vi "Q1.vi"() -> ()   [LabVIEW 2019]
uses:
  <vilib>/measure/matone.llb/Extract Multiple Tone Information 1 Chan.vi
  <vilib>/measure/matone.llb/Extract Single Tone Information N Chan.vi
  <vilib>/measure/NI_MAPro.lvlib
panel:
  out "DHT <=10%":bool[](array[boolean])
  in  "stop":bool
  in  "LIGAR":bool
  in  "file path":path=path "C:/lista2.tdms"
  out "ONDA TOTAL":waveform(dbl)(graph)
  out "multiple tone information":T1(array[cluster]) {"detected phase (deg)" format="%_6g"; "detected amplitude" format="%_6p"; "detected frequency" format="%_6p"}
  out "ONDA 1":dynamicdata(graph)
  out "ONDA 3":dynamicdata(graph)
  out "ONDA 2":dynamicdata(graph)
  out "ONDA 4":dynamicdata(graph)
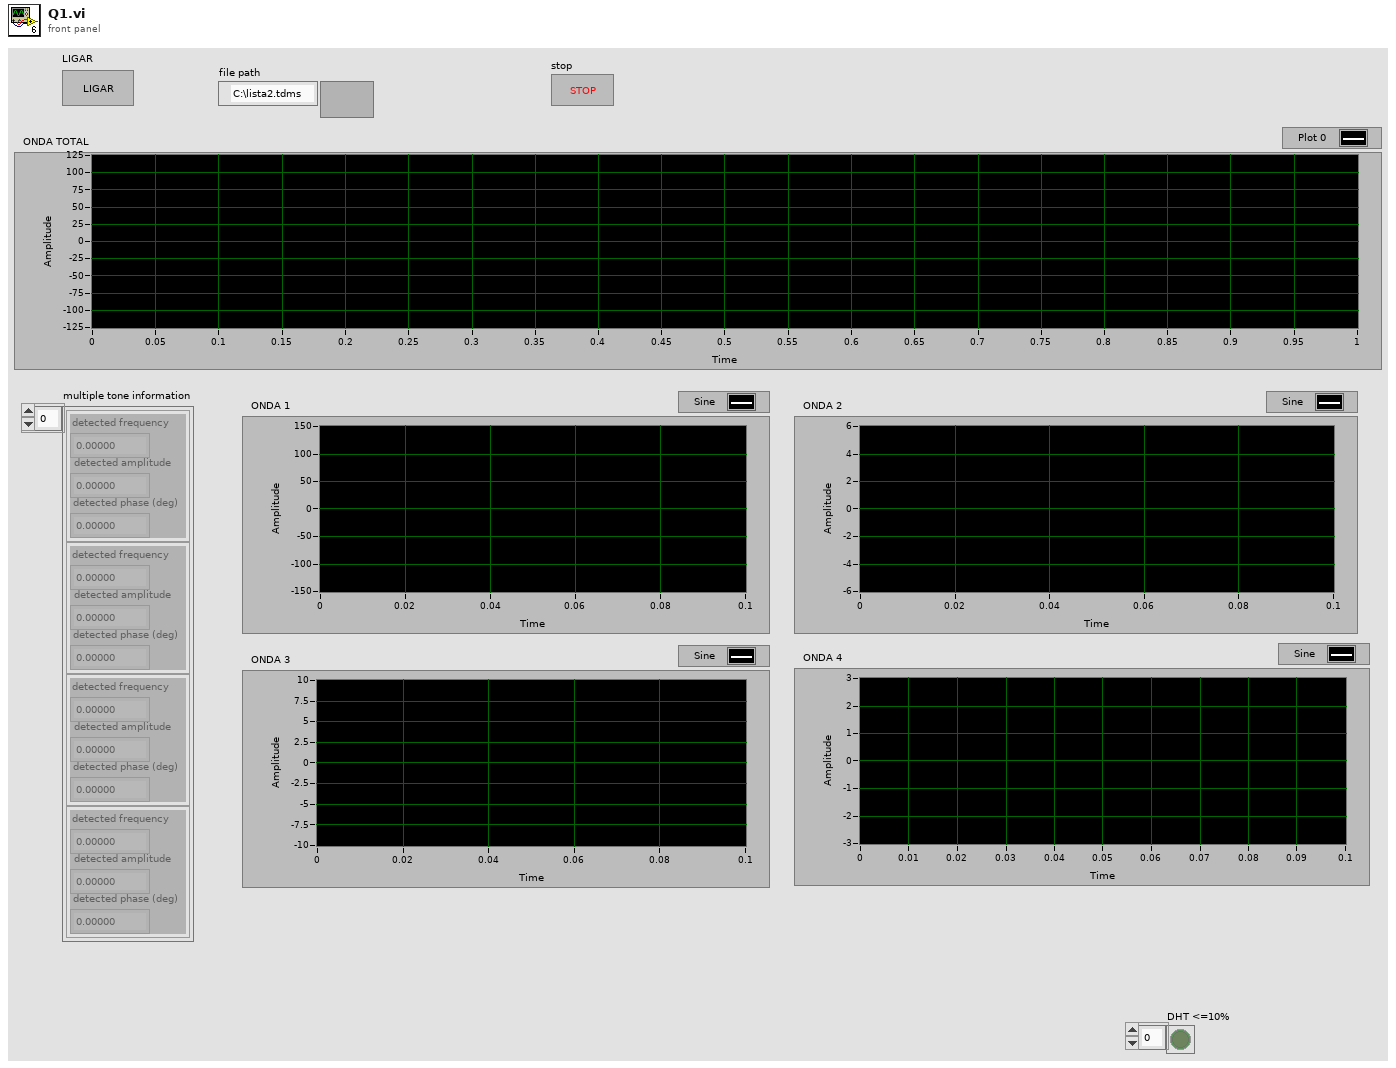
[diagram p1: front panel]
types:
  T1 = cluster{"detected frequency":dbl, "detected amplitude":dbl, "detected phase (deg)":dbl}[]
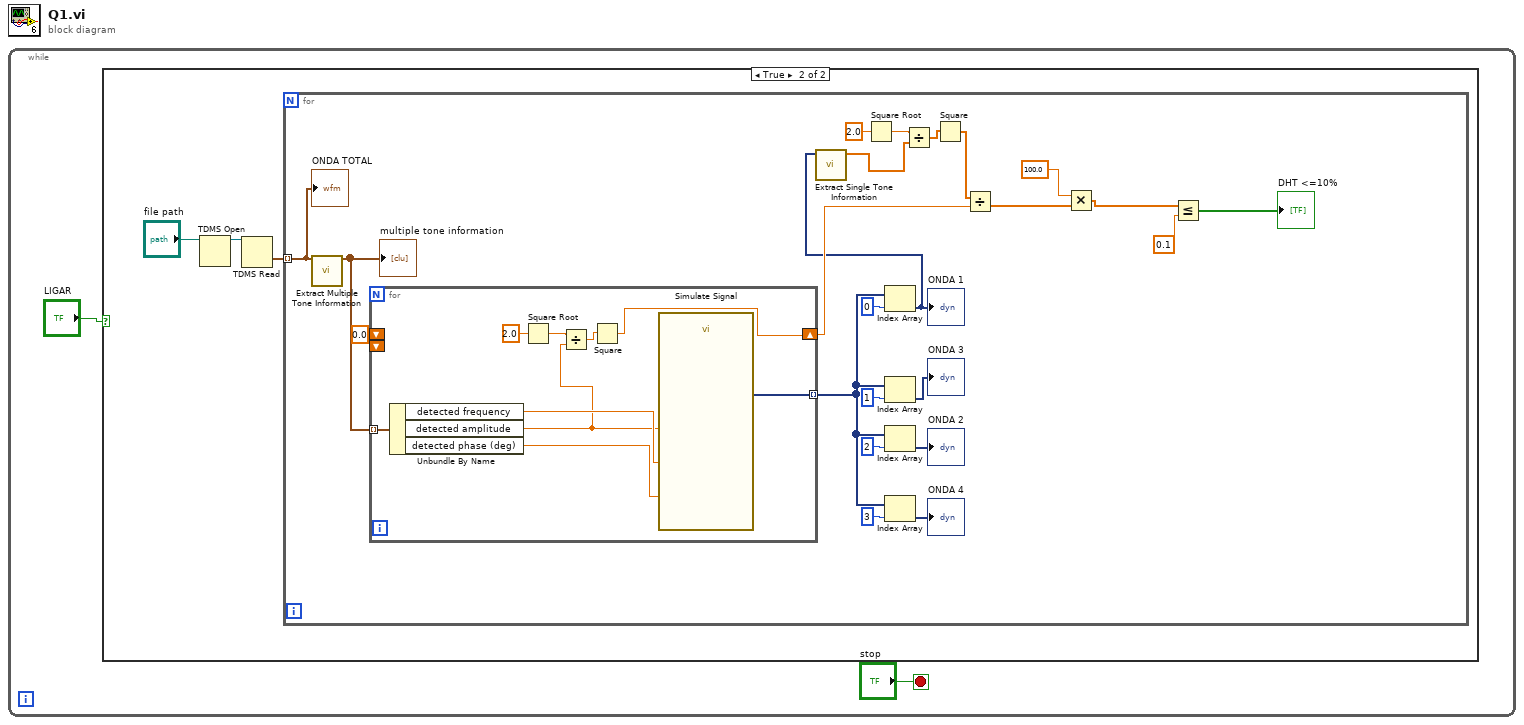
[diagram p0: block diagram]
diagram:
  n1 = while {
    stop <- "stop" stop-if-true
    n2 = case shown="True" "LIGAR" {
      frame False {
      }
      frame True {
        n3 = TDMS Open(11:"file path") -> (3:w4:refnum<k34>)  [unwired: 6 in, 1 out]
        n4 = TDMS Read(0:w4) -> (10:w3:waveform(dbl)[])  [unwired: 7 in, 5 out]
        n5 = for {
          tunnel: w3 -> [w28] mode=indexing
          w18 = 0.0 ("detected amplitude")
          n6 = call-poly <vilib>:"Extract Multiple Tone Information.vi"("time signal in"=w28) -> ("multiple tone information"=w27:T1)  [unwired: 12 in, 2 out]
          "multiple tone information" <- w27
          n7 = for {
            tunnel: w27 -> [w37] mode=indexing
            tunnel: [w35] -> w19 mode=indexing
            shift-right: [w33] -> w17
            shift-left: w18 -> [_]
            shift-left: w18 -> [_]
            n8 = Unbundle By Name(w37) -> ("detected frequency"=w36:dbl, "detected amplitude"=w30:dbl, "detected phase (deg)"=w34:dbl)
            n9 = Square Root(x=2.0) -> (sqrt(x)=w31:dbl)
            n10 = Divide(x=w31, y=w30) -> (x/y=w29:dbl)
            n11 = Square(x=w29) -> (x^2=w33:dbl)
            n12 = call "Simulate Signal"("Frequency"=w36, "Amplitude"=w30, "Phase"=w34) -> ("Sine"=w35:dynamicdata)  [unwired: 11 in, 1 out]
          }
          n13 = Square Root(x=2.0) -> (sqrt(x)=w13:dbl)
          n14 = Index Array(array=w19, index=0) -> (element=w16:dynamicdata)
          "ONDA 1" <- w16
          n15 = call-poly <vilib>:"Extract Single Tone Information.vi"("time signals in"=w16) -> ("detected frequencies"=w11:dbl[])  [unwired: 5 in, 5 out]
          n16 = Index Array(array=w19, index=1) -> (element=→"ONDA 3":dynamicdata)
          n17 = Index Array(array=w19, index=2) -> (element=→"ONDA 2":dynamicdata)
          n18 = Index Array(array=w19, index=3) -> (element=→"ONDA 4":dynamicdata)
          n19 = Divide(x=w13, y=w11) -> (x/y=w12:dbl[])
          n20 = Square(x=w12) -> (x^2=w10:dbl[])
          n21 = Divide(x=w10, y=w17) -> (x/y=w9:dbl[])
          n22 = Multiply(x=100.0, y=w9) -> (x*y=w7:dbl[])
          n23 = Less Or Equal?(x=w7, y=0.1 ("x")) -> (x <= y?=→"DHT <=10%":bool[])
          "ONDA TOTAL" <- w28
        }
      }
    }
  }
